vi "Example.vi"() -> ()   [LabVIEW 2025]
uses:
  console_debug.dll
panel:
  in  "arg1":string
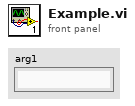
[diagram p1: front panel]
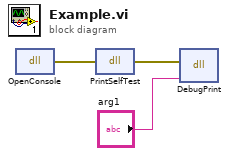
[diagram p0: block diagram]
diagram:
  n1 = dll-call lib="C:/Users/vboxuser/Documents/RUST/DebugConsole/console_debug.dll" fn="OpenConsole"() -> (error out=w3:errorcluster)  [unwired: 4 in, 1 out]
  n2 = dll-call lib="C:/Users/vboxuser/Documents/RUST/DebugConsole/console_debug.dll" fn="PrintSelfTest"(error in=w3) -> (error out=w2:errorcluster)  [unwired: 3 in, 1 out]
  n3 = dll-call lib="C:/Users/vboxuser/Documents/RUST/DebugConsole/console_debug.dll" fn="DebugPrint"(error in=w2, "arg1"="arg1") -> ()  [unwired: 4 in, 2 out]
